vi "Install Support_Pre-Install Custom Action.vi"(10 "Variant":variant) -> (0 "error out":errorcluster)   [LabVIEW 2021]
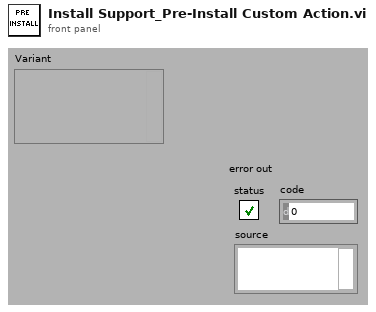
[diagram p1: front panel]
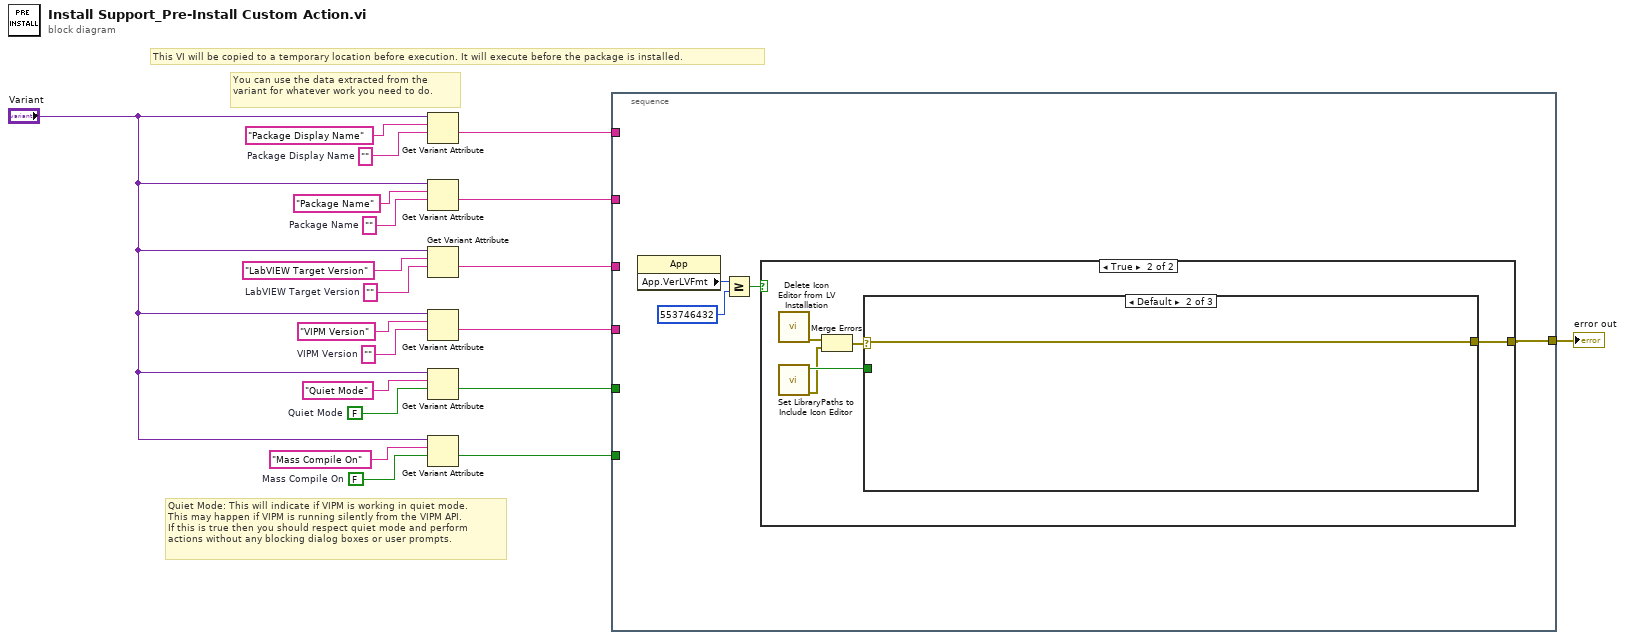
[diagram p0: block diagram]
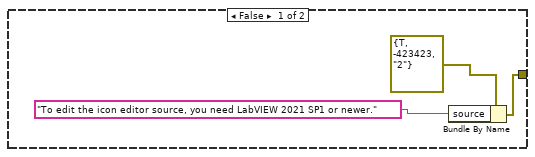
[diagram p2: hidden frame]
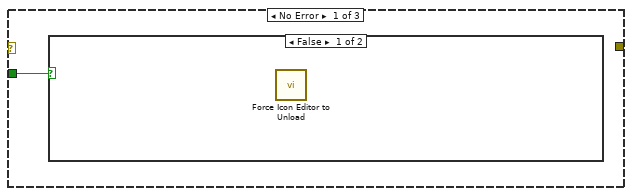
[diagram p3: hidden frame]
diagram:
  w2 = FALSE  # Mass Compile On
  w4 = ""  # Package Display Name
  w11 = FALSE  # Quiet Mode
  w14 = ""  # VIPM Version
  w16 = ""  # LabVIEW Target Version
  w18 = ""  # Package Name
  # "You can use the data extracted from the variant for whatever work you need to do."
  # "Quiet Mode: This will indicate if VIPM is working in quiet mode.\nThis may happen if VIPM is running silently from the VIPM API.\nIf this is true then you should respect quiet mode and perform\nactions without any blocking dialog boxes or user prompts."
  # "This VI will be copied to a temporary location before execution. It will execute before the package is installed."
  n1 = Get Variant Attribute(Variant="Variant", name="Package Display Name", default value (empty Variant)=w4) -> (value=w10:string)  [unwired: 1 in, 3 out]
  n2 = Get Variant Attribute(Variant="Variant", name="Package Name", default value (empty Variant)=w18) -> (value=w9:string)  [unwired: 1 in, 3 out]
  n3 = Get Variant Attribute(Variant="Variant", name="LabVIEW Target Version", default value (empty Variant)=w16) -> (value=w8:string)  [unwired: 1 in, 3 out]
  n4 = Get Variant Attribute(Variant="Variant", name="VIPM Version", default value (empty Variant)=w14) -> (value=w7:string)  [unwired: 1 in, 3 out]
  n5 = Get Variant Attribute(Variant="Variant", name="Quiet Mode", default value (empty Variant)=w11) -> (value=w6:bool)  [unwired: 1 in, 3 out]
  n6 = Get Variant Attribute(Variant="Variant", name="Mass Compile On", default value (empty Variant)=w2) -> (value=w5:bool)  [unwired: 1 in, 3 out]
  n7 = stacked-sequence {
    tunnel: w10 -> [_]
    tunnel: w9 -> [_]
    tunnel: w8 -> [_]
    tunnel: w7 -> [_]
    tunnel: w6 -> [_]
    tunnel: w5 -> [_]
    tunnel: [w21] -> w1
    frame #0 {
      n8 = property class="App"() -> ("App.VerLVFmt"=w24:i32)  [unwired: 2 in, 2 out]
      n9 = Greater Or Equal?(x=w24, y=553746432 ("Application:Version As Integer")) -> (x >= y?=w22:bool)
      n10 = case shown="True" w22 {
        tunnel: [w26 w28] -> w21
        frame False {
          n11 = Bundle By Name(cluster=errorcluster {"status"=TRUE, "code"=-423423, "source"="2"} ("error IO"), "source"="To edit the icon editor source, you need LabVIEW 2021 SP1 or newer." ("message")) -> (w26:errorcluster)
        }
        frame True {
          n12 = call "Delete Icon Editor from LV Installation.vi"() -> ("error out"=w31:errorcluster)  [unwired: 10 in, 1 out]
          n13 = call "Set LibraryPaths to Include Icon Editor.vi"() -> ("error out"=w29:errorcluster, "config modified?"=w32:bool)  [unwired: 10 in]
          n14 = Merge Errors(w31, w29) -> (w30:errorcluster)
          n15 = case shown="Default" w30 {
            selector: w30 -> [_ w34 w35]
            tunnel: w32 -> [w33 _ _]
            tunnel: [_ w34 w35] -> w28
            frame No Error {
              n16 = case shown="False" w33 {
                frame False {
                  n17 = call "Force Icon Editor to Unload.vi"() -> ()  [unwired: 12 in]
                }
                frame True {
                }
              }
            }
            frame Default {
            }
            frame Error {
              # "User cancelled, no further interaction needed"
            }
          }
        }
      }
    }
  }
  "error out" <- w1
